vi "DetectElectroMan.vi"(8 "error in (no error)":errorcluster caption="错误输入（无错误）") -> (0 "error out":errorcluster caption="错误输出")   [LabVIEW 2014, in "DetectElectros.lvlib"]
uses:
  DetectElectros.lvlib
  <vilib>/Utility/miscctls.llb/LVRowAndColumnTypeDef.ctl
  DataBase/DataBase.lvlib
panel:
  out "area_name0":string
  out "一行记录":string[](array[string])
  out "结果字符串":string
  in  "OK":bool
  in  "退出":bool
  in  "预览":bool
  in  "清空":bool
  in  "修改":bool
  in  "删除按钮":bool
  in  "添加按钮":bool
  in  "检测电极":i32(listbox)
  in  "填埋区域":i32(listbox)
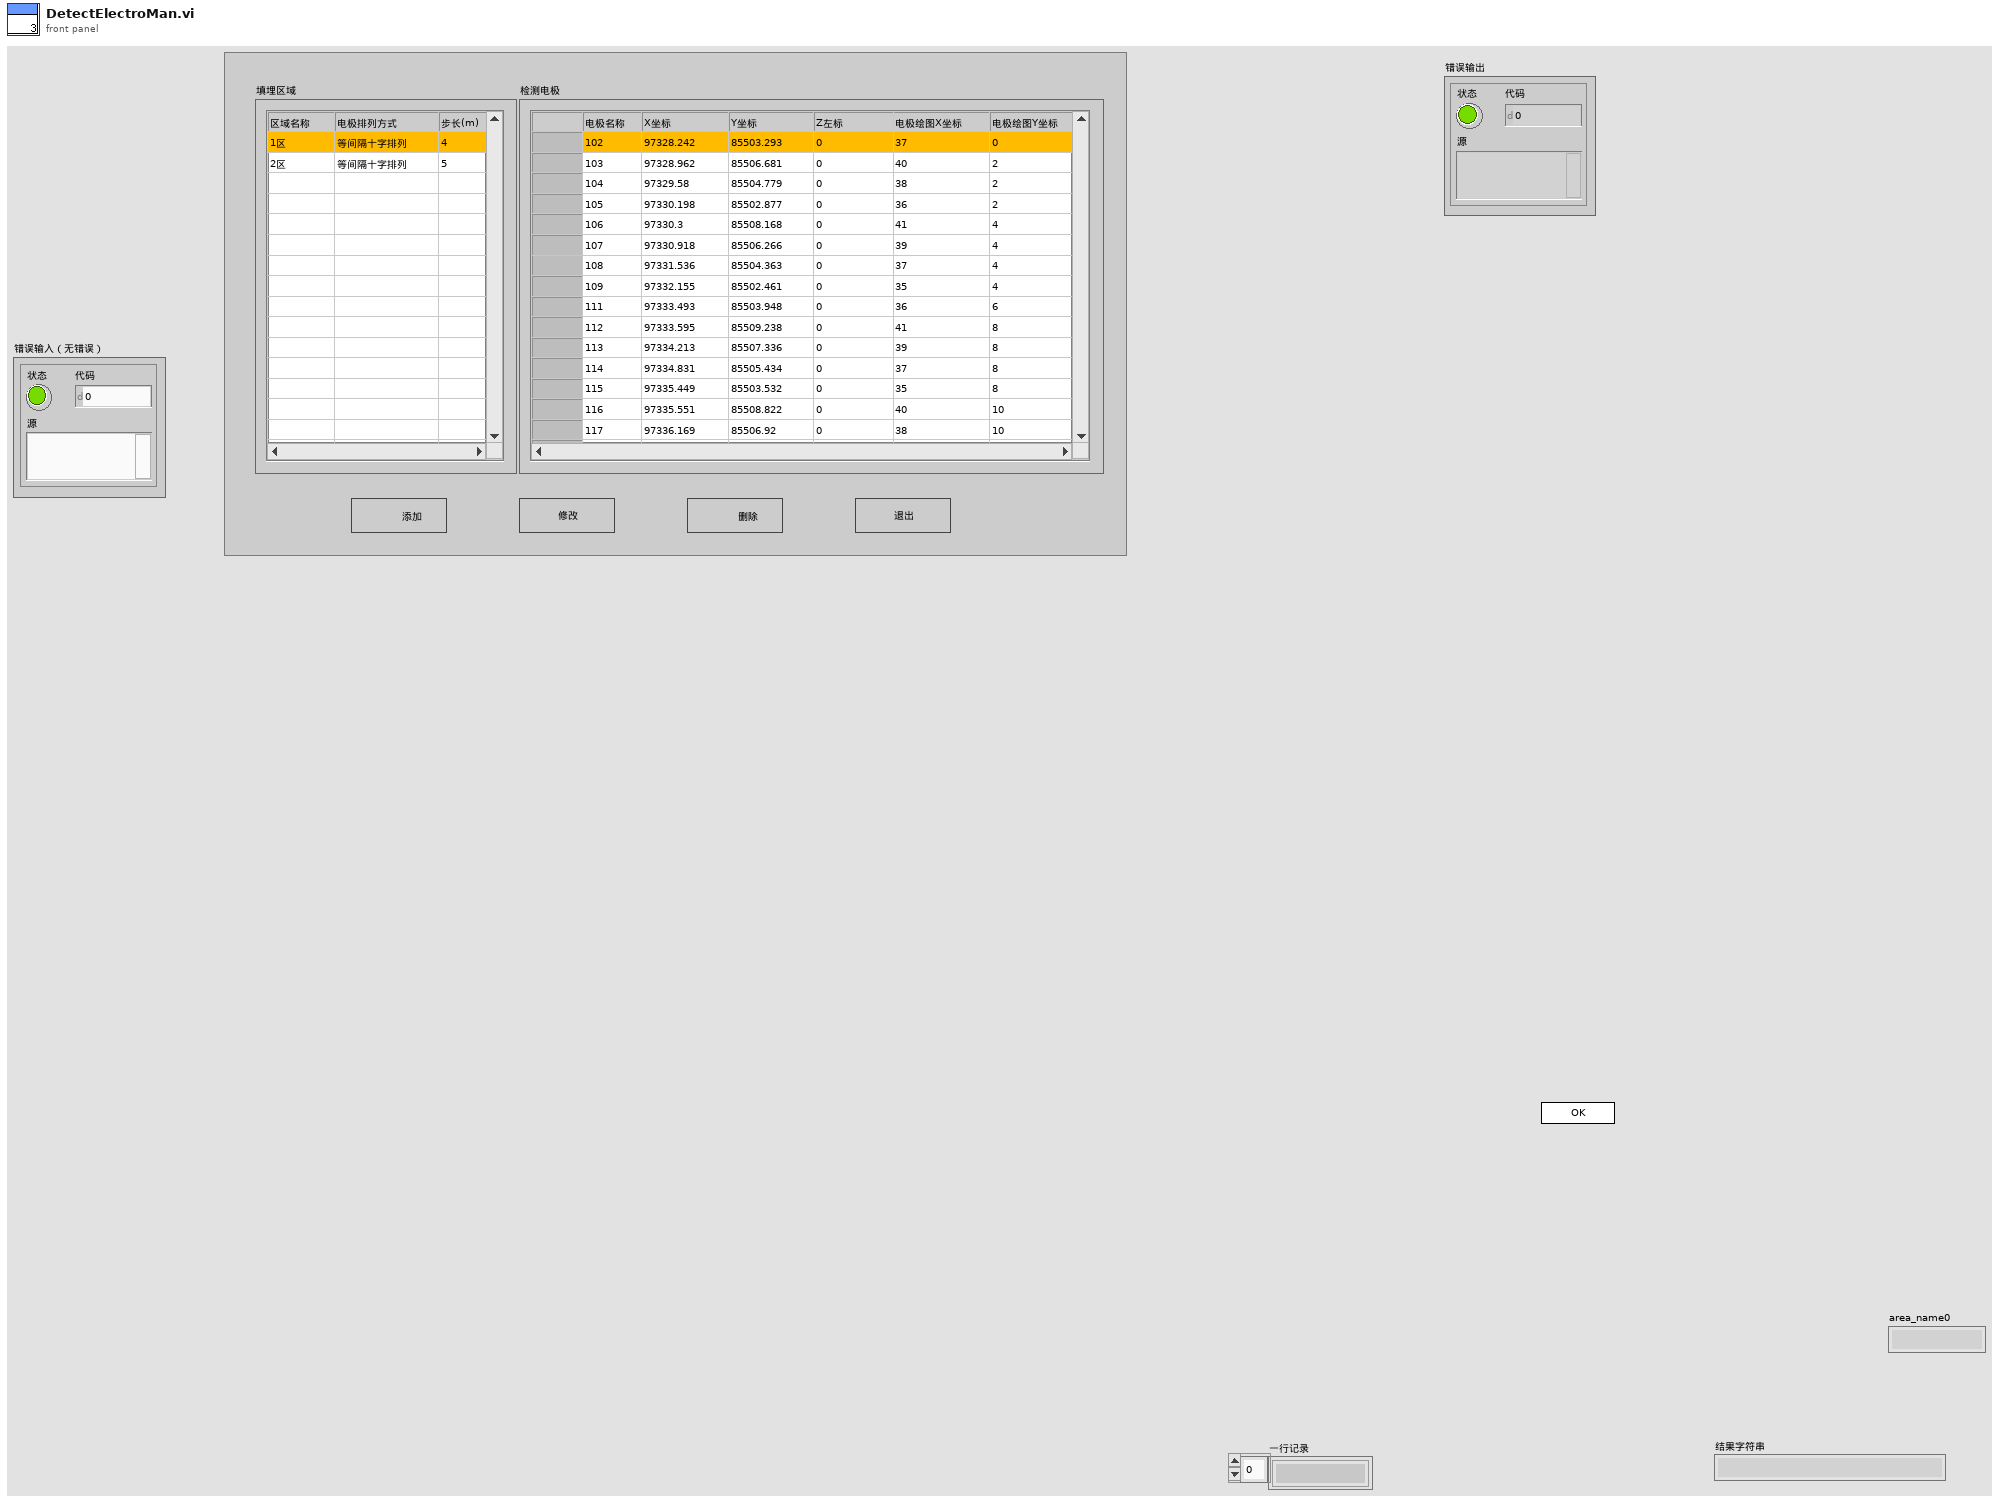
[diagram p1: front panel]
types:
  T1 = enum32{"invalid app kind", "Development System", "Run Time System", "Student Edition", "Embedded LabVIEW", "Evaluation", "Custom"}
  T2 = enum32{"Invalid", "Standard", "Closed", "Hidden", "Minimized", "Maximized"}
  T3 = typedef "LVPoint32TypeDef.ctl" = cluster{"Horizontal":i32, "Vertical":i32}
  T4 = typedef "LVRowAndColumnTypeDef.ctl" = cluster{"Row":i32, "Column":i32}
  T5 = cluster{"Core":cluster{"Current VI Reference":refnum<vi>, "Close Panel on Exit?":bool}, "Your Boolean data":bool, "Your string data":string, "填埋区行列D":T4, "area_name":string, "检测电极行列D":T4}
  T6 = cluster{"Current VI Reference":refnum<vi>, "Close Panel on Exit?":bool}
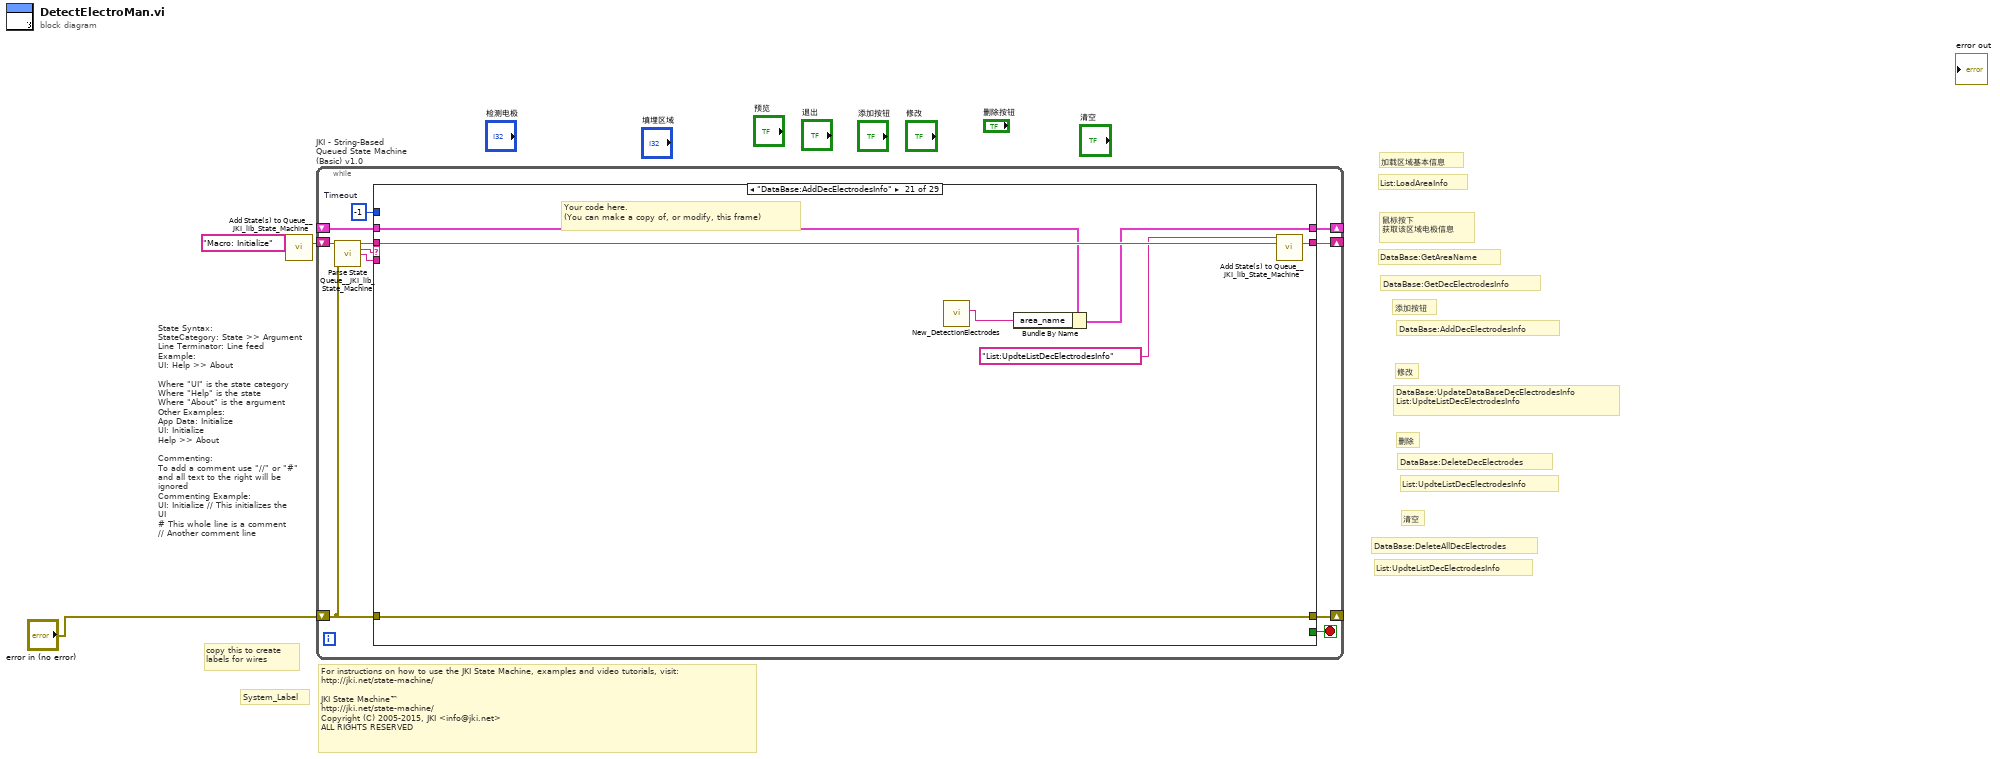
[diagram p0: block diagram]
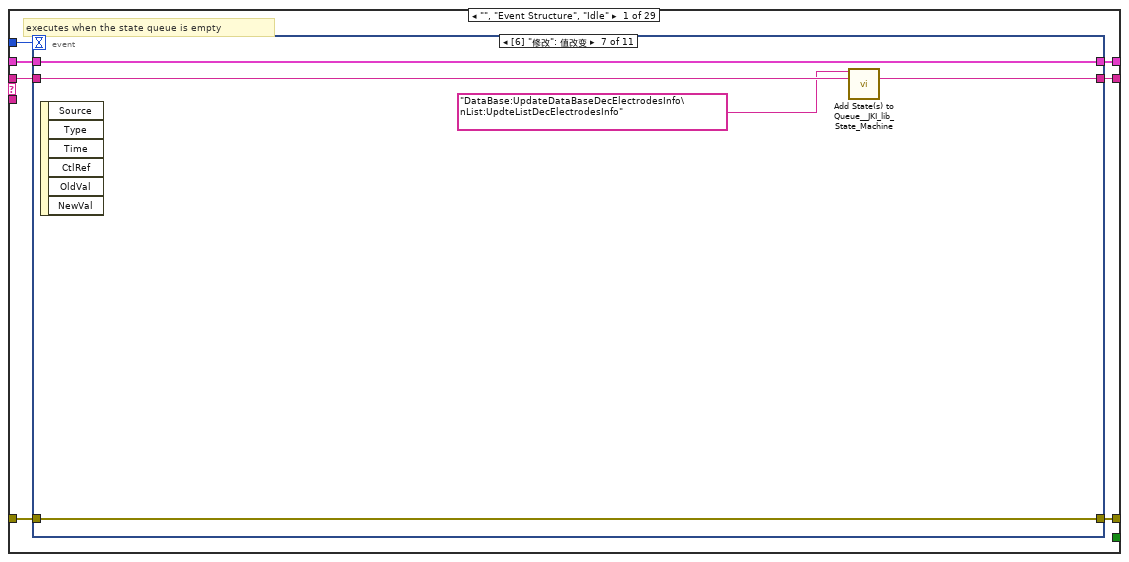
[diagram p2: hidden frame]
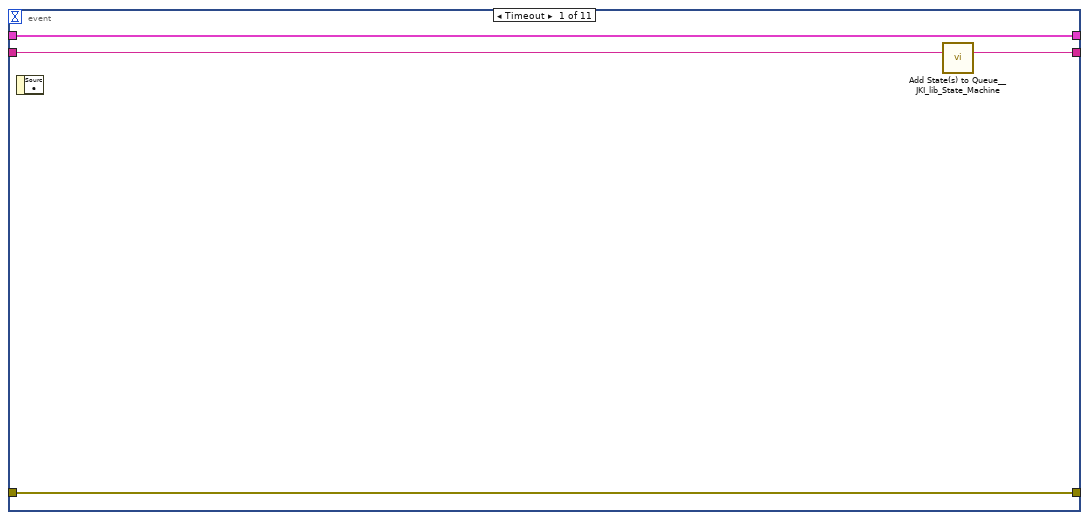
[diagram p3: hidden frame]
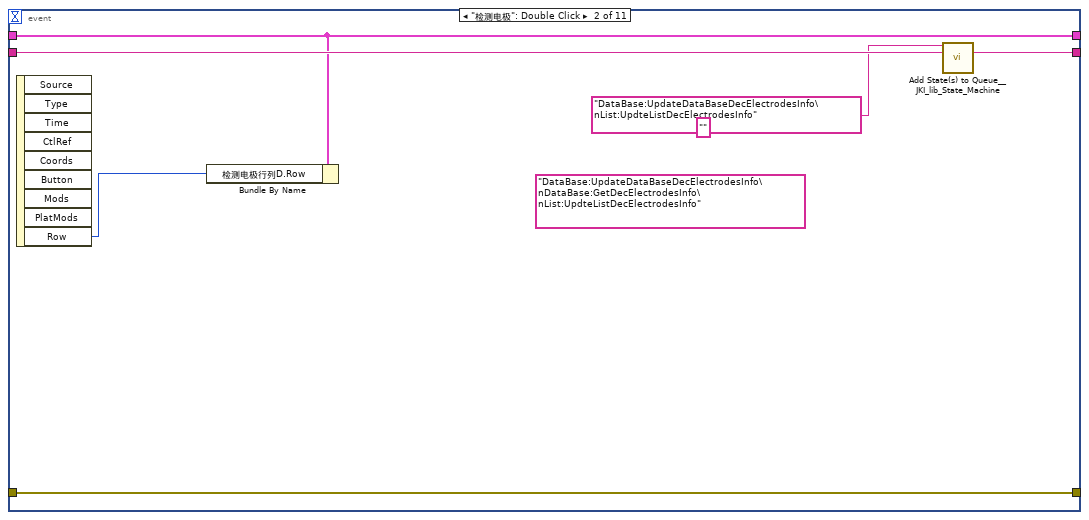
[diagram p4: hidden frame]
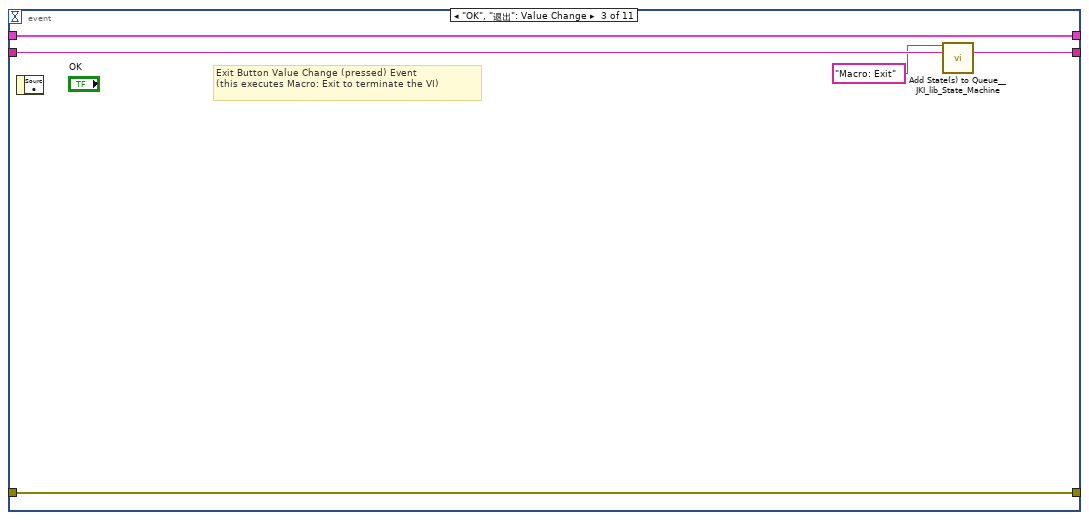
[diagram p5: hidden frame]
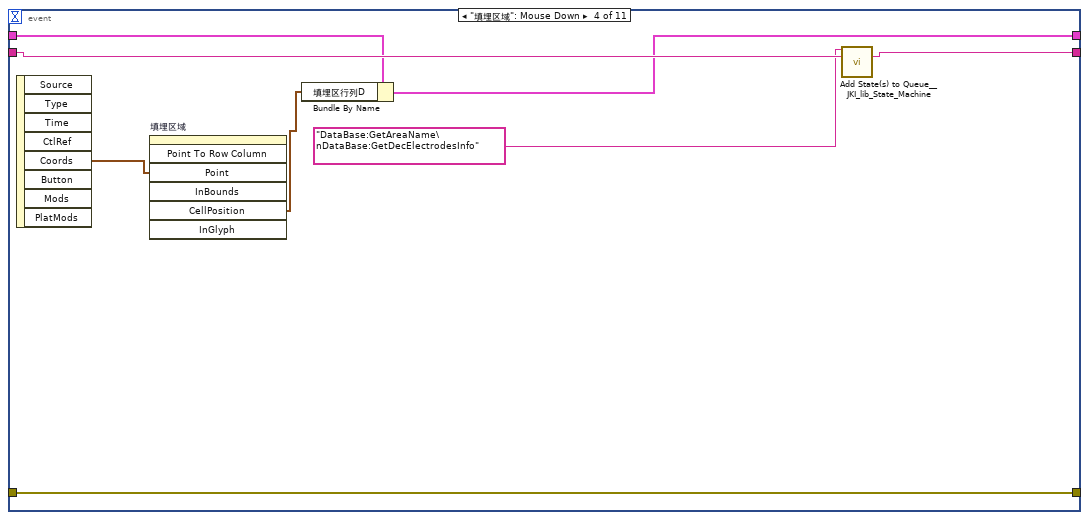
[diagram p6: hidden frame]
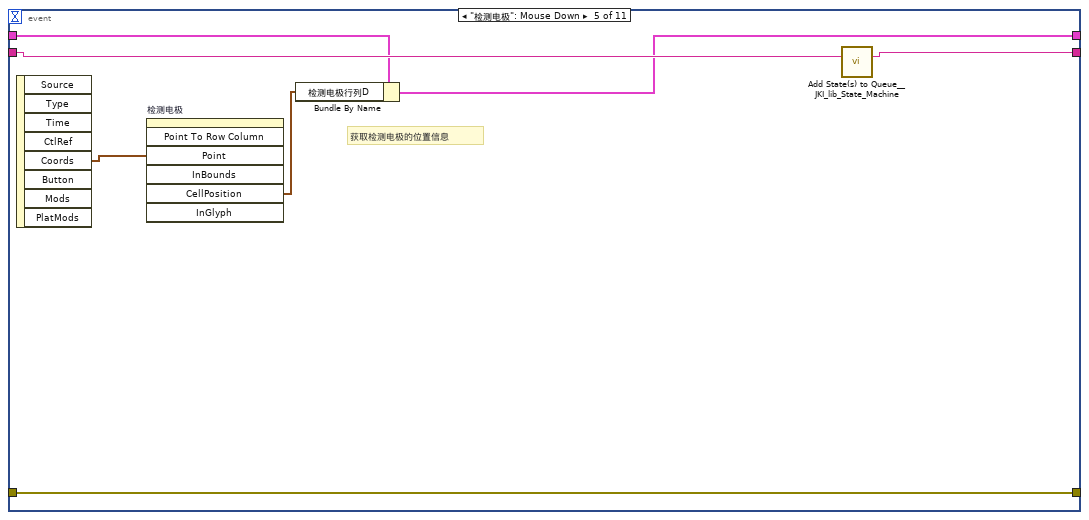
[diagram p7: hidden frame]
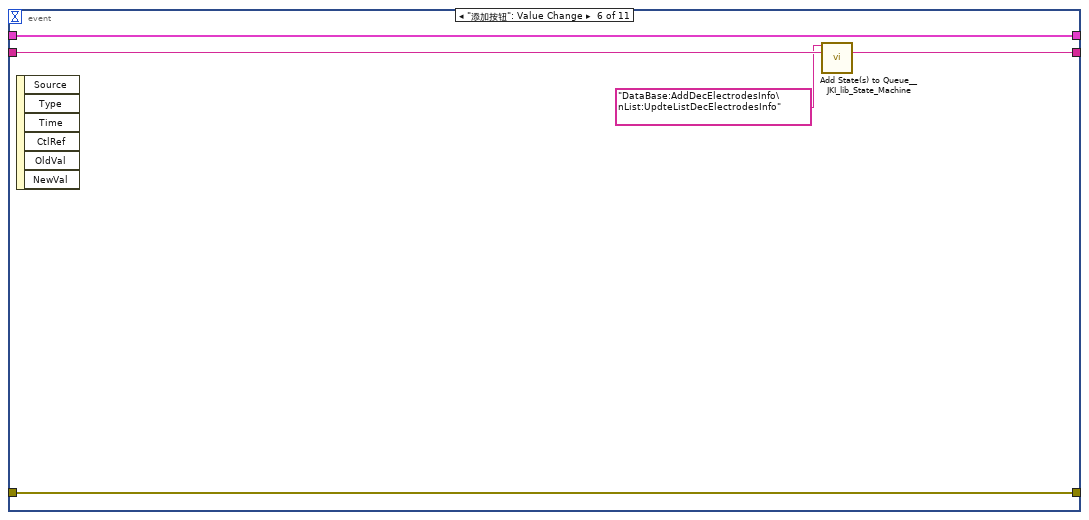
[diagram p8: hidden frame]
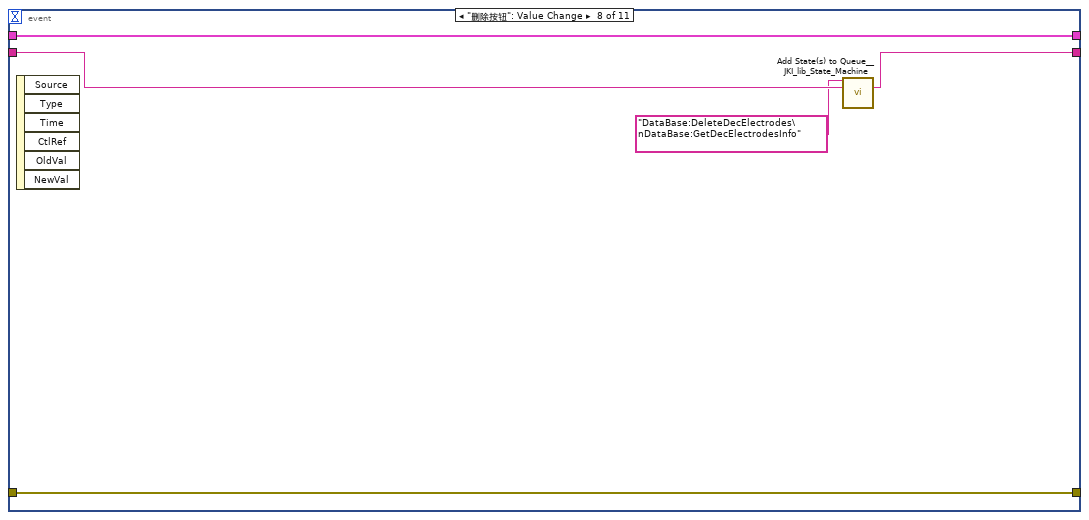
[diagram p9: hidden frame]
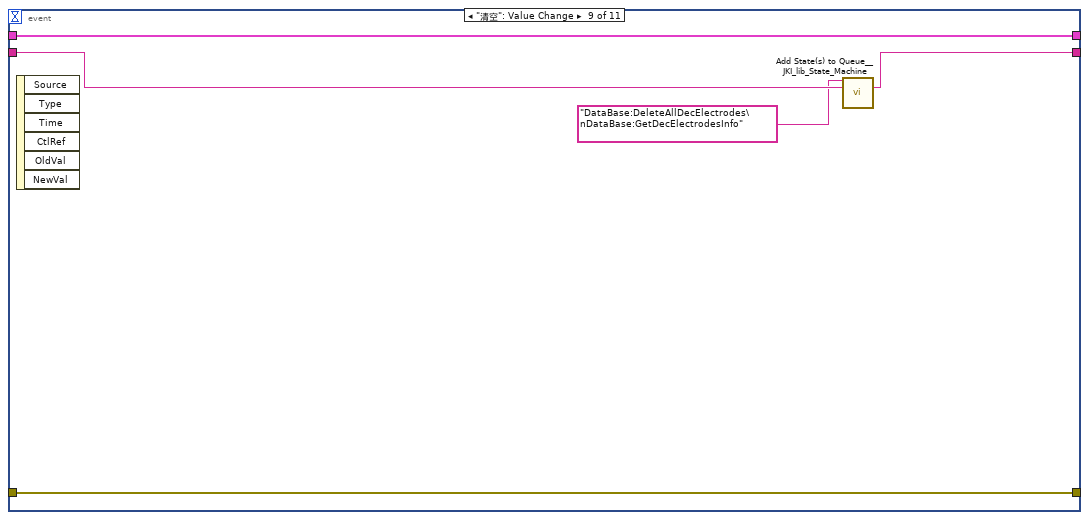
[diagram p10: hidden frame]
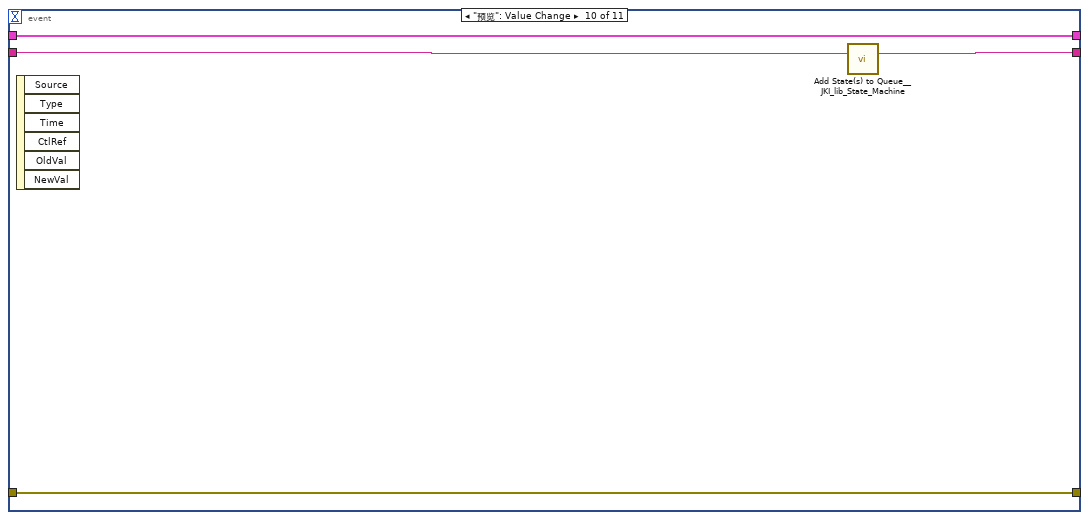
[diagram p11: hidden frame]
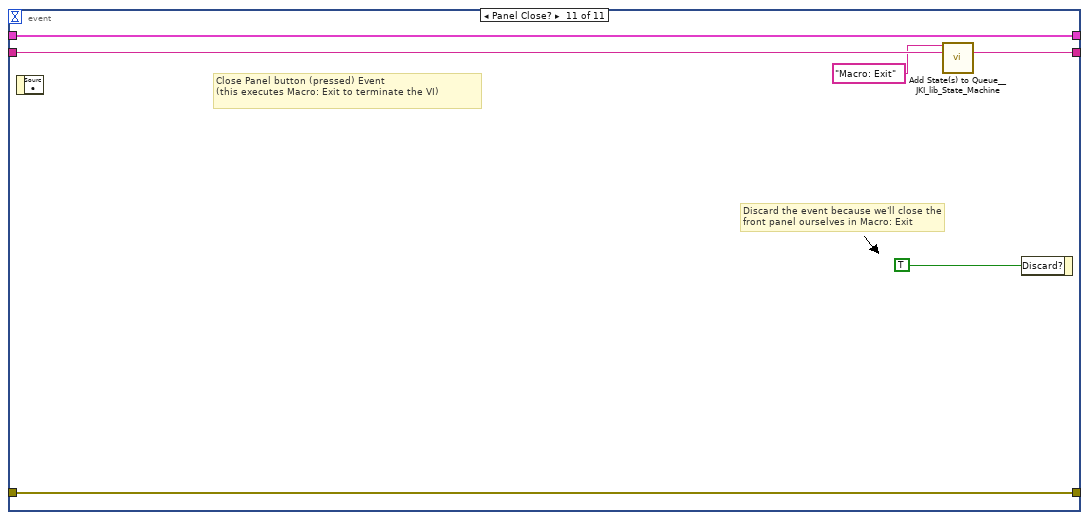
[diagram p12: hidden frame]
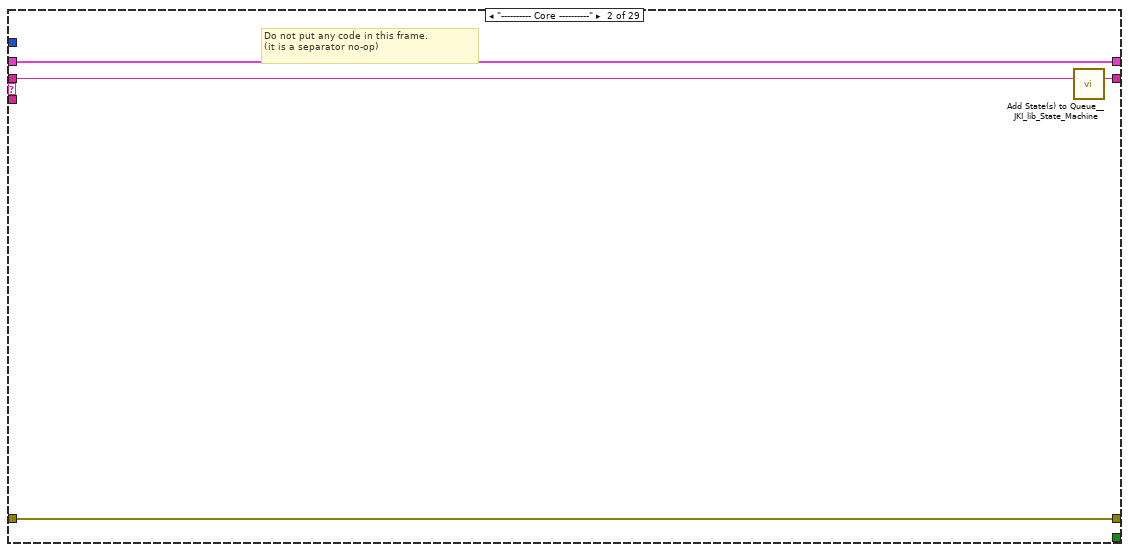
[diagram p13: hidden frame]
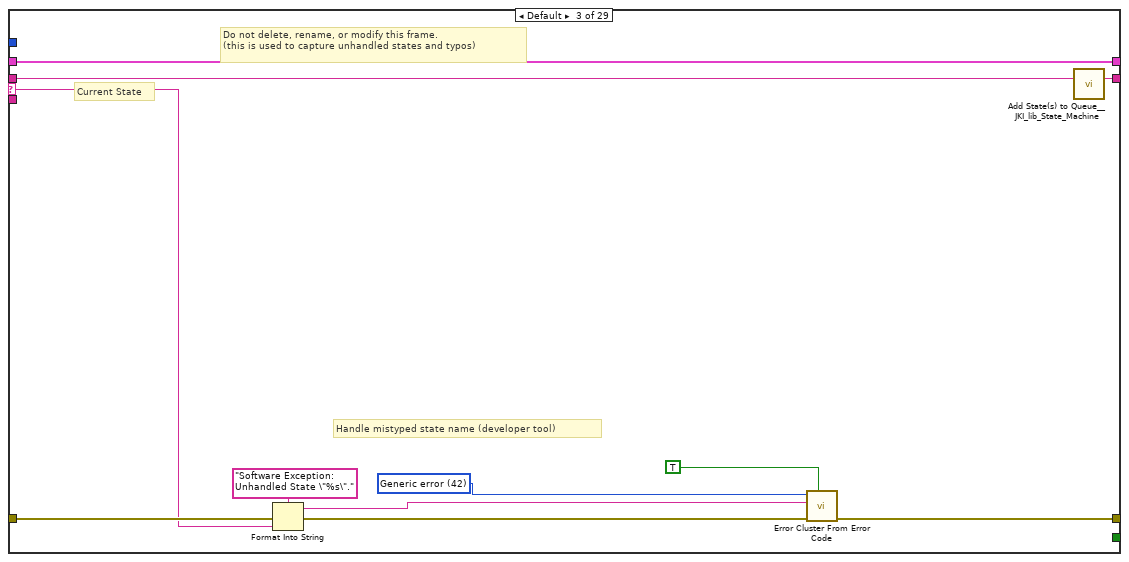
[diagram p14: hidden frame]
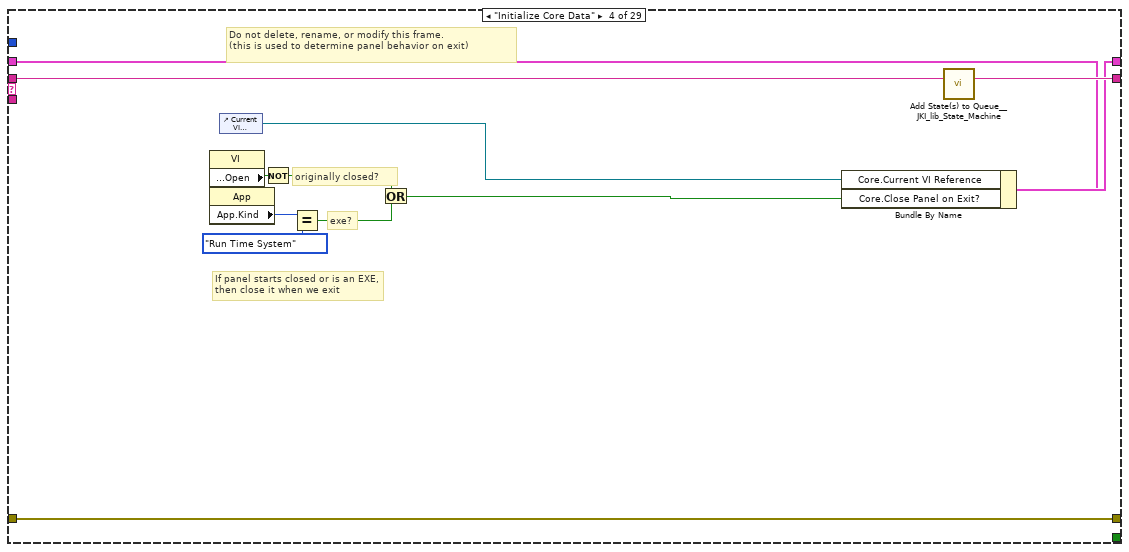
[diagram p15: hidden frame]
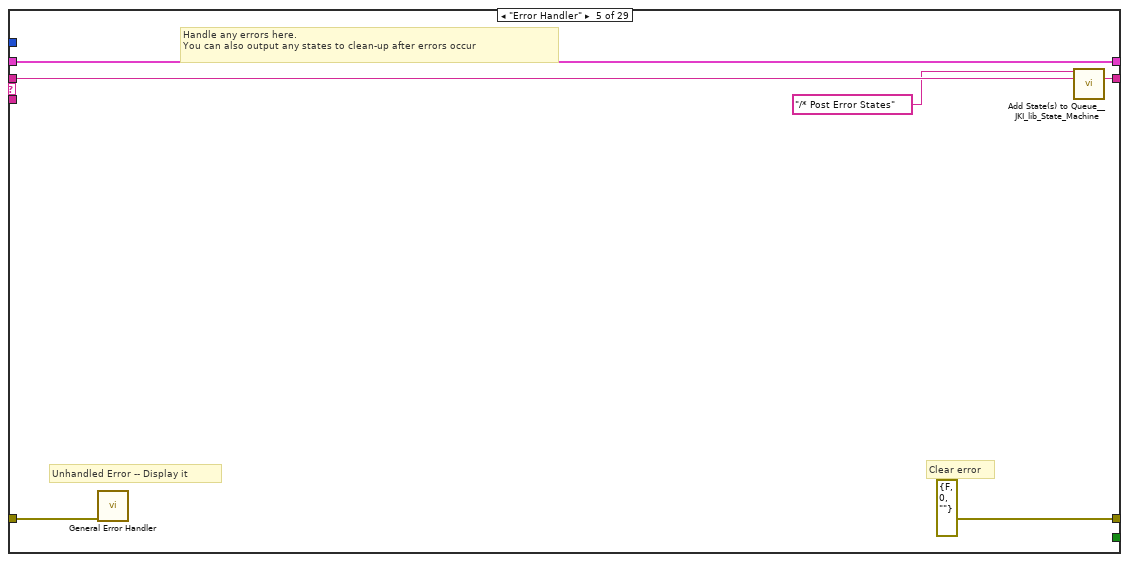
[diagram p16: hidden frame]
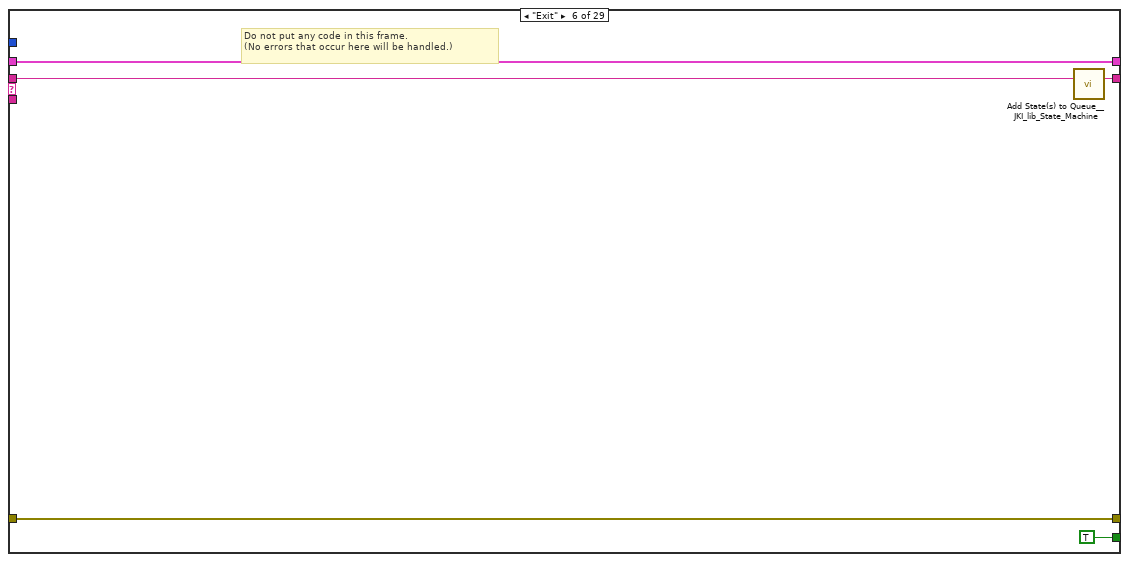
[diagram p17: hidden frame]
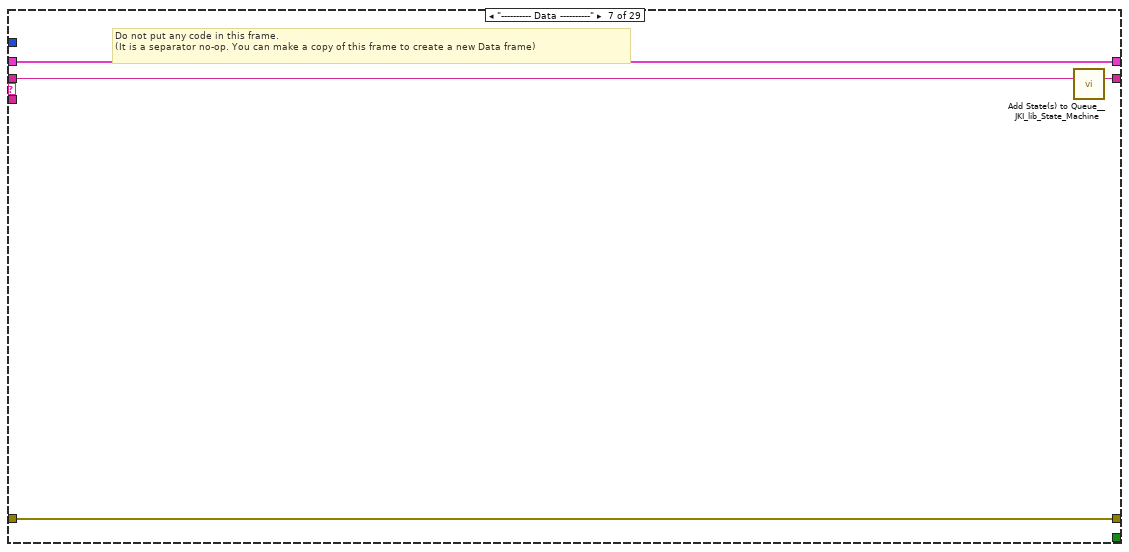
[diagram p18: hidden frame]
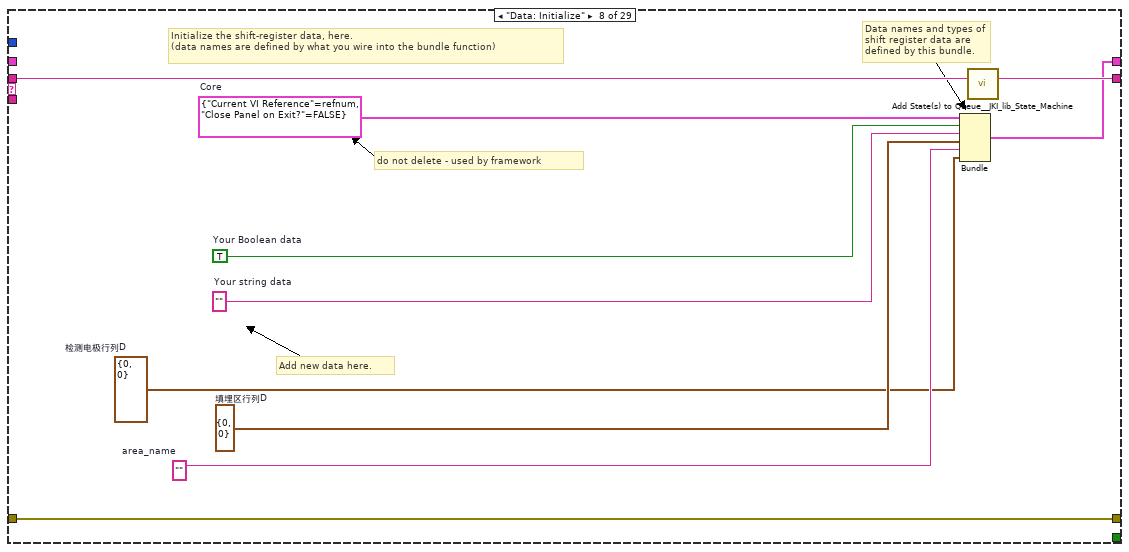
[diagram p19: hidden frame]
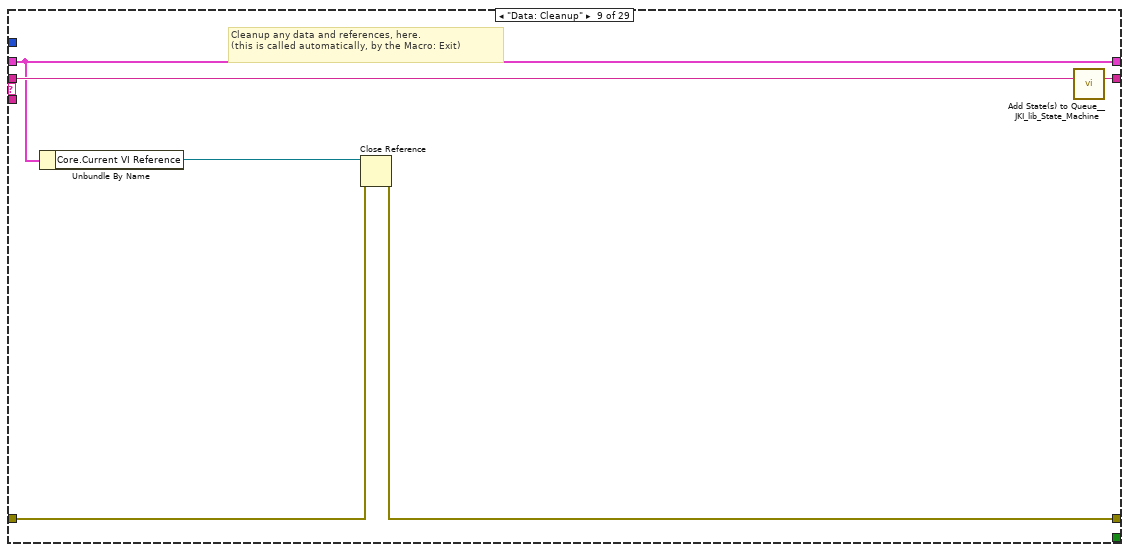
[diagram p20: hidden frame]
diagram:
  # "DataBase:AddDecElectrodesInfo"
  # "添加按钮"
  # "List:UpdteListDecElectrodesInfo"
  # "DataBase:DeleteAllDecElectrodes"
  # "清空"
  # "List:UpdteListDecElectrodesInfo"
  # "DataBase:GetAreaName"
  # "DataBase:DeleteDecElectrodes"
  # "删除"
  # "DataBase:UpdateDataBaseDecElectrodesInfo\nList:UpdteListDecElectrodesInfo"
  # "修改"
  # "DataBase:GetDecElectrodesInfo"
  # "鼠标按下\n获取该区域电极信息"
  # "List:LoadAreaInfo"
  # "加载区域基本信息"
  # "For instructions on how to use the JKI State Machine, examples and video tutorials, visit:\nhttp://jki.net/state-machine/\n\nJKI State Machine™\nhttp://jki.net/state-machine/\nCopyright (C) 2005-2015, JKI <info@jki.net>\nALL RIGHTS RESERVED"
  # "State Syntax:\nStateCategory: State >> Argument\nLine Terminator: Line feed\nExample:\nUI: Help >> About\n\nWhere \"UI\" is the state category\nWhere \"Help\" is the state\nWhere \"About\" is the argument\nOther Examples:\nApp Data: Initialize\nUI: Initialize\nHelp >> About\n\nCommenting:\nTo add a comment use \"//\" or \"#\" and all text to the right will be ignored\nCommenting Example:\nUI: Initialize // This initializes the UI\n# This whole line is a comment\n// Another comment line"
  # "copy this to create labels for wires"
  # "System_Label"
  n1 = call <vilib>:"Add State(s) to Queue__JKI_lib_State_Machine.vi"("State(s) in (\"\")"="Macro: Initialize") -> ("States Out"=w3:string)  [unwired: 14 in]
  n2 = while "JKI - String-Based Queued State Machine (Basic) v1.0" {
    shift-right: [w7] -> _
    shift-left: _ -> [w6]
    shift-right: [w10] -> _
    shift-left: "error in (no error)" -> [w4]
    shift-right: [w9] -> _
    shift-left: w3 -> [w11]
    stop <- w8 stop-if-true
    w5 = -1  # Timeout
    n3 = call <vilib>:"Parse State Queue__JKI_lib_State_Machine.vi"("State Queue"=w11, "Error In (no error)"=w4) -> ("Remaining States"=w13:string, "Current State"=w14:string, "Arguments"=w12:string)  [unwired: 11 in]
    n4 = case shown="\"DataBase:AddDecElectrodesInfo\"" w14 {
      selector: w14 -> [_ _ w86 _ _ _ _ _ _ _ _ _ _ _ _ _ _ _ _ _ _ _ _ _ _ _ _ _ _]
      tunnel: w13 -> [w21 w85 w90 w108 w114 w119 w123 w133 w139 w143 w148 w154 w165 w191 w196 w206 w210 w214 w218 w222 w229 w237 w254 w266 w275 w289 w293 w307 w316]
      tunnel: w12 -> [_ _ _ _ _ _ _ _ _ _ _ w149 w159 _ _ _ _ _ _ _ _ _ _ _ _ _ _ _ _]
      tunnel: w6 -> [w19 w82 w88 w99 w111 w117 w120 _ w134 w140 w146 w152 w161 w188 w193 w203 w207 w211 w215 w219 w225 w232 w239 w259 w268 w277 w290 w295 w313]
      tunnel: [w18 w83 w92 w105 errorcluster {"status"=FALSE, "code"=0, "source"=""} ("error out") w116 w121 w130 w135 w141 w145 w150 w162 w189 w194 w204 w208 w212 w216 w220 w227 w235 w252 w264 w273 w287 w291 w305 w314] -> w10
      tunnel: w4 -> [w17 w83 w91 w105 w110 w116 w121 w130 w136 w141 w145 w151 w163 w189 w194 w204 w208 w212 w216 w220 w227 w235 w252 w264 w273 w287 w291 w305 w314]
      tunnel: [w20 w84 w89 w107 w113 w118 w122 w132 w138 w142 w147 w153 w164 w190 w195 w205 w209 w213 w217 w221 w228 w236 w253 w265 w274 w288 w292 w306 w315] -> w9
      tunnel: [_ _ _ _ _ TRUE _ _ _ _ _ _ _ _ _ _ _ _ _ _ _ _ _ _ _ _ _ _ _] -> w8
      tunnel: [w16 w82 w88 w106 w111 w117 w120 w131 w134 w140 w146 w152 w161 w188 w193 w203 w207 w211 w215 w219 w224 w232 w238 w259 w267 w277 w290 w295 w313] -> w7
      tunnel: w5 -> [w15 _ _ _ _ _ _ _ _ _ _ _ _ _ _ _ _ _ _ _ _ _ _ _ _ _ _ _ _]
      frame "", "Event Structure", "Idle" {
        # "executes when the state queue is empty"
        n5 = event shown="[6] \"修改\": 值改变" {
          selector: _ -> [_ _ _ _ _ _ _ _ _ _ _]
          dyn-events: _ -> [_ _ _ _ _ _ _ _ _ _ _]
          timeout: w15 -> [_ _ _ _ _ _ _ _ _ _ _]
          tunnel: w21 -> [w25 w31 w36 w43 w50 w54 w60 w64 w69 w73 w81]
          tunnel: [w24 w30 w35 w44 w51 w55 w61 w65 w70 w74 w80] -> w20
          tunnel: w19 -> [w22 w28 w33 w39 w48 w56 w58 w66 w71 w75 w78]
          tunnel: [w23 w29 w34 w42 w49 w53 w59 w62 w67 w72 w79] -> w18
          tunnel: w17 -> [w23 w29 w34 w42 w49 w53 w59 w62 w67 w72 w79]
          tunnel: [w22 w28 w33 w38 w47 w56 w58 w66 w71 w75 w78] -> w16
          event Timeout {
            n6 = event-data() -> ()  [unwired: 1 in, 1 out]
            n7 = call <vilib>:"Add State(s) to Queue__JKI_lib_State_Machine.vi"("State(s) in (\"\")"=w25) -> ("States Out"=w24:string)  [unwired: 14 in]
          }
          event "检测电极": Double Click {
            (unwired) "DataBase:UpdateDataBaseDecElectrodesInfo\nDataBase:GetDecElectrodesInfo\nList:UpdteListDecElectrodesInfo"
            (unwired) ""
            n8 = event-data() -> ("Row"=w27:i32)  [unwired: 1 in, 8 out]
            n9 = Bundle By Name(cluster=w28, "检测电极行列D.Row"=w27) -> ()  [unwired: 1 out]
            n10 = call <vilib>:"Add State(s) to Queue__JKI_lib_State_Machine.vi"("State(s) in Front (\"\")"="DataBase:UpdateDataBaseDecElectrodesInfo\nList:UpdteListDecElectrodesInfo", "State(s) in (\"\")"=w31) -> ("States Out"=w30:string)  [unwired: 13 in]
          }
          event "OK", "退出": Value Change {
            # "Exit Button Value Change (pressed) Event\n(this executes Macro: Exit to terminate the VI)"
            n11 = event-data() -> ()  [unwired: 1 in, 1 out]
            n12 = call <vilib>:"Add State(s) to Queue__JKI_lib_State_Machine.vi"("State(s) in Front (\"\")"="Macro: Exit", "State(s) in (\"\")"=w36) -> ("States Out"=w35:string)  [unwired: 13 in]
          }
          event "填埋区域": Mouse Down {
            n13 = event-data() -> ("Coords"=w41:T3)  [unwired: 1 in, 7 out]
            n14 = invoke on="填埋区域" class="MCListbox (严格)" method="Point To Row Column"("Point"=w41) -> ("CellPosition"=w40:T4)  [unwired: 6 in, 6 out]
            n15 = Bundle By Name(cluster=w39, "填埋区行列D"=w40) -> (w38:T5)
            n16 = call <vilib>:"Add State(s) to Queue__JKI_lib_State_Machine.vi"("State(s) in Front (\"\")"="DataBase:GetAreaName\nDataBase:GetDecElectrodesInfo", "State(s) in (\"\")"=w43) -> ("States Out"=w44:string)  [unwired: 13 in]
          }
          event "检测电极": Mouse Down {
            # "获取检测电极的位置信息"
            n17 = event-data() -> ("Coords"=w46:T3)  [unwired: 1 in, 7 out]
            n18 = invoke on="检测电极" class="MCListbox (严格)" method="Point To Row Column"("Point"=w46) -> ("CellPosition"=w45:T4)  [unwired: 6 in, 6 out]
            n19 = Bundle By Name(cluster=w48, "检测电极行列D"=w45) -> (w47:T5)
            n20 = call <vilib>:"Add State(s) to Queue__JKI_lib_State_Machine.vi"("State(s) in (\"\")"=w50) -> ("States Out"=w51:string)  [unwired: 14 in]
          }
          event "添加按钮": Value Change {
            n21 = event-data() -> ()  [unwired: 1 in, 6 out]
            n22 = call <vilib>:"Add State(s) to Queue__JKI_lib_State_Machine.vi"("State(s) in Front (\"\")"="DataBase:AddDecElectrodesInfo\nList:UpdteListDecElectrodesInfo", "State(s) in (\"\")"=w54) -> ("States Out"=w55:string)  [unwired: 13 in]
          }
          event "修改": Value Change {
            n23 = event-data() -> ()  [unwired: 1 in, 6 out]
            n24 = call <vilib>:"Add State(s) to Queue__JKI_lib_State_Machine.vi"("State(s) in Front (\"\")"="DataBase:UpdateDataBaseDecElectrodesInfo\nList:UpdteListDecElectrodesInfo", "State(s) in (\"\")"=w60) -> ("States Out"=w61:string)  [unwired: 13 in]
          }
          event "删除按钮": Value Change {
            n25 = event-data() -> ()  [unwired: 1 in, 6 out]
            n26 = call <vilib>:"Add State(s) to Queue__JKI_lib_State_Machine.vi"("State(s) in Front (\"\")"="DataBase:DeleteDecElectrodes\nDataBase:GetDecElectrodesInfo", "State(s) in (\"\")"=w64) -> ("States Out"=w65:string)  [unwired: 13 in]
          }
          event "清空": Value Change {
            n27 = event-data() -> ()  [unwired: 1 in, 6 out]
            n28 = call <vilib>:"Add State(s) to Queue__JKI_lib_State_Machine.vi"("State(s) in Front (\"\")"="DataBase:DeleteAllDecElectrodes\nDataBase:GetDecElectrodesInfo", "State(s) in (\"\")"=w69) -> ("States Out"=w70:string)  [unwired: 13 in]
          }
          event "预览": Value Change {
            n29 = event-data() -> ()  [unwired: 1 in, 6 out]
            n30 = call <vilib>:"Add State(s) to Queue__JKI_lib_State_Machine.vi"("State(s) in (\"\")"=w73) -> ("States Out"=w74:string)  [unwired: 14 in]
          }
          event Panel Close? {
            # "Discard the event because we'll close the front panel ourselves in Macro: Exit"
            # "Close Panel button (pressed) Event\n(this executes Macro: Exit to terminate the VI)"
            n31 = event-data() -> ()  [unwired: 1 in, 1 out]
            n32 = call <vilib>:"Add State(s) to Queue__JKI_lib_State_Machine.vi"("State(s) in Front (\"\")"="Macro: Exit", "State(s) in (\"\")"=w81) -> ("States Out"=w80:string)  [unwired: 13 in]
            n33 = event-data("Discard?"=TRUE) -> ()  [unwired: 1 in, 1 out]
          }
        }
      }
      frame "---------- Core ----------" {
        # "Do not put any code in this frame.\n(it is a separator no-op)"
        n34 = call <vilib>:"Add State(s) to Queue__JKI_lib_State_Machine.vi"("State(s) in (\"\")"=w85) -> ("States Out"=w84:string)  [unwired: 14 in]
      }
      frame Default {
        w95 = 42 items=["No error", "Argument error", "Memory is full", "Out of zone", "End of file", "File already open", "Generic file I/O error", "File not found", "File permission error", "Disk is full", "Duplicate path", "Too many files open", "System feature not enabled", "Resource file not found", "Cannot add resource", "Resource not found", "Image not found", "Image memory error", "Pen does not exist", "Config type invalid", "Config token not found", "Config parse error", "Config memory error", "Bad external code format", "Bad external code offset", "External code not present", "Null window", "Destroy window error", "Null menu", "Print aborted", "Bad print record", "Print driver error", "Windows error during printing", "Memory error during printing", "Print dialog error", "Generic print error", "Invalid device refnum", "Device not found", "Device parameter error", "Device unit error", "Cannot open device", "Device call aborted", "Generic error", "Cancelled by user", "Object ID too low", "Object ID too high", "Object not in heap", "Unknown heap", "Unknown object (invalid DefProc)", "Unknown object (DefProc not in table)", "Message out of range", "Invalid (null) method", "Unknown message", "Manager call not supported", "Bad address", "Network operation in progress", "Network operation timed out", "Connection is busy", "Network attribute not supported", "Network error", "Address in use", "System out of memory", "Connection aborted", "Connection refused", "Not connected", "Already connected", "Connection closed", "Initialization error (interapplication manager)", "Bad occurrence", "Wait on unbound occurrence handler", "Occurrence queue overflow", "Datalog type conflict", "Unused", "Unrecognized type (interapplication manager)", "Memory corrupt", "Failed to make temporary DLL", "Old CIN version", "Drag socket not found", "Failed to load drop-object", "Failed to register OLE object", "Failed to release OLE object", "Format specifier type mismatch", "Unknown format specifier", "Too few format specifiers", "Too many format specifiers", "Scan failed", "Newer CIN version", "Error converting to variant", "Runtime menu error", "Password tampered", "Variant attribute not found", "Incompatible variant data type", "Event data is not available", "Event Store is not present", "Occurrence is not found", "Event Queue is not created", "Event info is not available", "Refnum passed is NULL", "Error retrieving Class GUID", "Error retrieving CoClass GUID", "Error retrieving TypeLib GUID.", "Bad built application magic bytes.", "Specific driver is different from the specific driver associated with the Logical Name.", "There is no session opened to the class driver.", "Max Error", "MAX - Error with config objects", "MAX - Error loading configuration", "MAX - Group not supported"]
        # "Current State"
        # "Do not delete, rename, or modify this frame.\n(this is used to capture unhandled states and typos)"
        # "Handle mistyped state name (developer tool)"
        n35 = Format Into String(format string="Software Exception: Unhandled State \"%s\"." ("message"), error in=w91, w86) -> (resulting string=w94:string, error out=w93:errorcluster)  [unwired: 1 in]
        n36 = call <vilib>:"Error Cluster From Error Code.vi"("show call chain? (False)"=TRUE, "error in (no error)"=w93, "error message (\"\")"=w94, "error code (0)"=w95) -> ("error out"=w92:errorcluster)  [unwired: 5 in]
        n37 = call <vilib>:"Add State(s) to Queue__JKI_lib_State_Machine.vi"("State(s) in (\"\")"=w90) -> ("States Out"=w89:string)  [unwired: 14 in]
      }
      frame "Initialize Core Data" {
        # "Do not delete, rename, or modify this frame.\n(this is used to determine panel behavior on exit)"
        # "originally closed?"
        # "exe?"
        # "If panel starts closed or is an EXE, then close it when we exit"
        n38 = property class="VI"() -> ("Front Panel.Open"=w104:bool)  [unwired: 2 in, 2 out]
        n39 = property class="App"() -> ("App.Kind"=w103:T1)  [unwired: 2 in, 2 out]
        n40 = control-ref of="Current VI Reference"() -> (w97:refnum<vi>)
        n41 = Not(x=w104) -> (.not. x?=w101:bool)
        n42 = Equal?(x=w103, y=T1."Run Time System" ("Application:Kind")) -> (x = y?=w100:bool)
        n43 = Or(x=w101, y=w100) -> (x .or. y?=w98:bool)
        n44 = Bundle By Name(cluster=w99, "Core.Current VI Reference"=w97, "Core.Close Panel on Exit?"=w98) -> (w106:T5)
        n45 = call <vilib>:"Add State(s) to Queue__JKI_lib_State_Machine.vi"("State(s) in (\"\")"=w108) -> ("States Out"=w107:string)  [unwired: 14 in]
      }
      frame "Error Handler" {
        # "Unhandled Error -- Display it"
        # "Handle any errors here.\nYou can also output any states to clean-up after errors occur"
        # "Clear error"
        n46 = call <vilib>:"General Error Handler.vi"("error in (no error)"=w110) -> ()  [unwired: 10 in, 5 out]
        n47 = call <vilib>:"Add State(s) to Queue__JKI_lib_State_Machine.vi"("State(s) in Front (\"\")"="/* Post Error States", "State(s) in (\"\")"=w114) -> ("States Out"=w113:string)  [unwired: 13 in]
      }
      frame "Exit" {
        # "Do not put any code in this frame.\n(No errors that occur here will be handled.)"
        n48 = call <vilib>:"Add State(s) to Queue__JKI_lib_State_Machine.vi"("State(s) in (\"\")"=w119) -> ("States Out"=w118:string)  [unwired: 14 in]
      }
      frame "---------- Data ----------" {
        # "Do not put any code in this frame.\n(It is a separator no-op. You can make a copy of this frame to create a new Data frame)"
        n49 = call <vilib>:"Add State(s) to Queue__JKI_lib_State_Machine.vi"("State(s) in (\"\")"=w123) -> ("States Out"=w122:string)  [unwired: 14 in]
      }
      frame "Data: Initialize" {
        w124 = T4 {"Row"=0, "Column"=0}  # 检测电极行列D
        w125 = ""  # area_name
        w126 = T4 {"Row"=0, "Column"=0}  # 填埋区行列D
        w127 = T6 {"Current VI Reference"=refnum, "Close Panel on Exit?"=FALSE}  # Core
        w129 = TRUE  # Your Boolean data
        w128 = ""  # Your string data
        # "do not delete - used by framework"
        # "Add new data here."
        # "Data names and types of shift register data are defined by this bundle."
        # "Initialize the shift-register data, here.\n(data names are defined by what you wire into the bundle function)"
        n50 = Bundle("Core"=w127, "Your Boolean data"=w129, "Your string data"=w128, "填埋区行列D"=w126, "area_name"=w125, "检测电极行列D"=w124) -> (w131:T5)  [unwired: 1 in]
        n51 = call <vilib>:"Add State(s) to Queue__JKI_lib_State_Machine.vi"("State(s) in (\"\")"=w133) -> ("States Out"=w132:string)  [unwired: 14 in]
      }
      frame "Data: Cleanup" {
        # "Cleanup any data and references, here.\n(this is called automatically, by the Macro: Exit)"
        n52 = Unbundle By Name(w134) -> ("Core.Current VI Reference"=w137:refnum<vi>)
        n53 = Close Reference(reference=w137, error in (no error)=w136) -> (error out=w135:errorcluster)
        n54 = call <vilib>:"Add State(s) to Queue__JKI_lib_State_Machine.vi"("State(s) in (\"\")"=w139) -> ("States Out"=w138:string)  [unwired: 14 in]
      }
      frame "---------- UI ----------" {
        # "Do not put any code in this frame.\n(It is a separator no-op. You can make a copy of this frame to create a new UI frame)"
        n55 = call <vilib>:"Add State(s) to Queue__JKI_lib_State_Machine.vi"("State(s) in (\"\")"=w143) -> ("States Out"=w142:string)  [unwired: 14 in]
      }
      frame "UI: Initialize" {
        # "Initialize the User Interface, here.\n(this is called automatically, by the Macro: Init)"
        n56 = call <vilib>:"Add State(s) to Queue__JKI_lib_State_Machine.vi"("State(s) in Front (\"\")"="List:LoadAreaInfo", "State(s) in (\"\")"=w148) -> ("States Out"=w147:string)  [unwired: 13 in]
      }
      frame "UI: Cursor Set" {
        # "Argument"
        # "Set and Unset Cursor Busy.\n(Usage: \"UI: Cursor Set >> Busy|Idle\")"
        n57 = case shown="\"Idle\", 默认" w149 {
          tunnel: w151 -> [w156 w158]
          tunnel: [w155 w157] -> w150
          frame "Idle", Default {
            n58 = call <vilib>:"Unset Busy.vi"("error in (no error)"=w156) -> ("error out"=w155:errorcluster)  [unwired: 10 in]
          }
          frame "Busy" {
            n59 = call <vilib>:"Set Busy.vi"("error in (no error)"=w158) -> ("error out"=w157:errorcluster)  [unwired: 9 in, 1 out]
          }
        }
        n60 = call <vilib>:"Add State(s) to Queue__JKI_lib_State_Machine.vi"("State(s) in (\"\")"=w154) -> ("States Out"=w153:string)  [unwired: 14 in]
      }
      frame "UI: Front Panel State" {
        # "Argument"
        # "Set Front Panel Open or Closed\n(Usage: \"UI: Front Panel State >> Open|Close\")"
        n61 = Unbundle By Name(w161) -> ("Core.Current VI Reference"=w160:refnum<vi>)
        n62 = case shown="\"Open\", 默认" w159 {
          tunnel: w163 -> [w169 w182]
          tunnel: [w171 w183] -> w162
          tunnel: w160 -> [w170 w180]
          frame "Open", Default {
            n63 = property class="VI"(reference=w170, error in=w169) -> (reference out=w167:refnum<vi>, error out=w168:errorcluster, "Front Panel.Open"=w166:bool)
            n64 = case shown="假" w166 {
              tunnel: [w174 w177] -> w171
              tunnel: w168 -> [w173 w177]
              tunnel: w167 -> [w172 _]
              frame False {
                n65 = invoke class="VI" method="FP.Open"(reference=w172, error in=w173, "Activate"=TRUE, "State"=T2."Standard") -> (error out=w174:errorcluster)  [unwired: 1 in, 4 out]
              }
              frame True {
              }
            }
          }
          frame "Close" {
            n66 = property class="VI"(reference=w180, error in=w182) -> (reference out=w179:refnum<vi>, error out=w181:errorcluster, "Front Panel.Open"=w178:bool)
            n67 = case shown="真" w178 {
              tunnel: [w184 w187] -> w183
              tunnel: w181 -> [w184 w186]
              tunnel: w179 -> [_ w185]
              frame False {
              }
              frame True {
                n68 = invoke class="VI" method="FP.Close"(reference=w185, error in=w186) -> (error out=w187:errorcluster)  [unwired: 1 in, 2 out]
              }
            }
          }
        }
        n69 = call <vilib>:"Add State(s) to Queue__JKI_lib_State_Machine.vi"("State(s) in (\"\")"=w165) -> ("States Out"=w164:string)  [unwired: 14 in]
      }
      frame "---------- Macro ----------" {
        # "Do not put any code in this frame.\n(It is a separator no-op. You can make a copy of this frame to create a new Macro frame)"
        n70 = call <vilib>:"Add State(s) to Queue__JKI_lib_State_Machine.vi"("State(s) in (\"\")"=w191) -> ("States Out"=w190:string)  [unwired: 14 in]
      }
      frame "Macro: Initialize" {
        w192 = "Data: Initialize\nInitialize Core Data\nUI: Initialize\nUI: Front Panel State >> Open"  # Data: Initialize Initialize Core Data UI: Initialize UI: Front Panel State >> Open
        # "Initialization Macro\n(This is called once, when the VI starts)"
        n71 = call <vilib>:"Add State(s) to Queue__JKI_lib_State_Machine.vi"("State(s) in Front (\"\")"=w192, "State(s) in (\"\")"=w196) -> ("States Out"=w195:string)  [unwired: 13 in]
      }
      frame "Macro: Exit" {
        # "Exit Macro\n(This is called once, when the VI exits)"
        n72 = Unbundle By Name(w203) -> ("Core.Close Panel on Exit?"=w202:bool)
        n73 = Select(t="UI: Front Panel State >> Close", s=w202, f="") -> (s? t:f=w199:string)
        n74 = call <vilib>:"Add State(s) to Queue__JKI_lib_State_Machine.vi"("State(s) in (\"\")"=w199, "State(s) at Back (\"\")"="Data: Cleanup\nExit") -> ("States Out"=w197:string)  [unwired: 13 in]
        n75 = call <vilib>:"Add State(s) to Queue__JKI_lib_State_Machine.vi"("State(s) in Front (\"\")"=w197, "State(s) in (\"\")"=w206) -> ("States Out"=w205:string)  [unwired: 13 in]
      }
      frame "---------- New Category ----------" {
        # "Template Separator\n(You can make a copy of, or modify, this frame)"
        n76 = call <vilib>:"Add State(s) to Queue__JKI_lib_State_Machine.vi"("State(s) in (\"\")"=w210) -> ("States Out"=w209:string)  [unwired: 14 in]
      }
      frame "New Category: 1" {
        # "Your code here.\n(You can make a copy of, or modify, this frame)"
        n77 = call <vilib>:"Add State(s) to Queue__JKI_lib_State_Machine.vi"("State(s) in (\"\")"=w214) -> ("States Out"=w213:string)  [unwired: 14 in]
      }
      frame "New Category: 2" {
        # "Your code here.\n(You can make a copy of, or modify, this frame)"
        n78 = call <vilib>:"Add State(s) to Queue__JKI_lib_State_Machine.vi"("State(s) in (\"\")"=w218) -> ("States Out"=w217:string)  [unwired: 14 in]
      }
      frame "----------DataBase----------" {
        # "Your code here.\n(You can make a copy of, or modify, this frame)"
        n79 = call <vilib>:"Add State(s) to Queue__JKI_lib_State_Machine.vi"("State(s) in (\"\")"=w222) -> ("States Out"=w221:string)  [unwired: 14 in]
      }
      frame "DataBase:AddDecElectrodesInfo" {
        # "Your code here.\n(You can make a copy of, or modify, this frame)"
        n80 = call "New_DetectionElectrodes.vi"() -> ("AreaName"=w226:string)  [unwired: 11 in]
        n81 = Bundle By Name(cluster=w225, "area_name"=w226) -> (w224:T5)
        n82 = call <vilib>:"Add State(s) to Queue__JKI_lib_State_Machine.vi"("State(s) in Front (\"\")"="List:UpdteListDecElectrodesInfo", "State(s) in (\"\")"=w229) -> ("States Out"=w228:string)  [unwired: 13 in]
      }
      frame "DataBase:DeleteAllDecElectrodes" {
        # "Your code here.\n(You can make a copy of, or modify, this frame)"
        n83 = Unbundle By Name(w232) -> ("area_name"=w231:string)
        n84 = Format Into String(format string="delete from t_detection_electrodes where  area_name='%s';", w231) -> (resulting string=w234:string)  [unwired: 2 in, 1 out]
        n85 = call "deleteData.vi"("SQL query"=w234) -> ()  [unwired: 10 in, 1 out]
        n86 = call <vilib>:"Add State(s) to Queue__JKI_lib_State_Machine.vi"("State(s) in Front (\"\")"="List:UpdteListDecElectrodesInfo", "State(s) in (\"\")"=w237) -> ("States Out"=w236:string)  [unwired: 13 in]
      }
      frame "DataBase:GetAreaName" {
        # "Your code here.\n(You can make a copy of, or modify, this frame)"
        n87 = Unbundle By Name(w239) -> ("填埋区行列D.Row"=w251:i32)
        n88 = Absolute Value(x=w251) -> (abs(x)=w242:i32)
        n89 = Number To Decimal String(number=w242) -> (decimal integer string=w248:string)  [unwired: 1 in]
        n90 = Format Into String(format string="select area_name from t_area limit %s,1;", w248) -> (resulting string=w249:string, error out=w247:errorcluster)  [unwired: 2 in]
        "结果字符串" <- w249
        n91 = call "SelectData.vi"("SQL query"=w249, "error in"=w247) -> ("recordset data"=w246:variant[][])  [unwired: 6 in, 1 out]
        n92 = call "ReadDataFromDatabase.vi"("长度"=1, "index"=0, "recordset data"=w246) -> ("一行记录"=w243:string[])  [unwired: 7 in, 1 out]
        "一行记录" <- w243
        n93 = Index Array(array=w243, index=0 ("索引")) -> (element=w240:string)
        "area_name0" <- w240
        n94 = Bundle By Name(cluster=w239, "area_name"=w240) -> (w238:T5)
        n95 = call <vilib>:"Add State(s) to Queue__JKI_lib_State_Machine.vi"("State(s) in (\"\")"=w254) -> ("States Out"=w253:string)  [unwired: 14 in]
      }
      frame "DataBase:DeleteDecElectrodes" {
        # "Your code here.\n(You can make a copy of, or modify, this frame)"
        n96 = Unbundle By Name(w259) -> ("检测电极行列D.Row"=w263:i32)
        n97 = Unbundle By Name(w259) -> ("area_name"=w258:string)
        n98 = Absolute Value(x=w263) -> (abs(x)=w261:i32)
        n99 = Number To Decimal String(number=w261) -> (decimal integer string=w260:string)  [unwired: 1 in]
        n100 = Format Into String(format string="delete from t_detection_electrodes where  detection_electrodes_id=(select td.detection_electrodes_id from (select detection_electrodes_id from t_detection_electrodes where  area_name='%s' limit %s,1) td);", w258, w260) -> (resulting string=w257:string, error out=w256:errorcluster)  [unwired: 2 in]
        n101 = call "deleteData.vi"("error in"=w256, "SQL query"=w257) -> ()  [unwired: 9 in, 1 out]
        n102 = call <vilib>:"Add State(s) to Queue__JKI_lib_State_Machine.vi"("State(s) in Front (\"\")"="List:UpdteListDecElectrodesInfo", "State(s) in (\"\")"=w266) -> ("States Out"=w265:string)  [unwired: 13 in]
      }
      frame "DataBase:UpdateDataBaseDecElectrodesInfo" {
        (unwired) "List:UpdteListDecElectrodesInfo"
        # "Your code here.\n(You can make a copy of, or modify, this frame)"
        n103 = Unbundle By Name(w268) -> ("area_name"=w270:string)
        n104 = Unbundle By Name(w268) -> ("检测电极行列D.Row"=w272:i32)
        n105 = Absolute Value(x=w272) -> (abs(x)=w271:i32)
        n106 = call "Modify_DetectionElectrodes.vi"("序号"=w271, "区域名称"=w270) -> ("out区域名称"=w269:string)  [unwired: 7 in, 2 out]
        n107 = Bundle By Name(cluster=w268, "area_name"=w269) -> (w267:T5)
        n108 = call <vilib>:"Add State(s) to Queue__JKI_lib_State_Machine.vi"("State(s) in (\"\")"=w275) -> ("States Out"=w274:string)  [unwired: 14 in]
      }
      frame "DataBase:GetDecElectrodesInfo" {
        # "Your code here.\n(You can make a copy of, or modify, this frame)"
        n109 = Unbundle By Name(w277) -> ("area_name"=w276:string)
        n110 = Format Into String(format string="select * from t_detection_electrodes where area_name='%s';", w276) -> (resulting string=w285:string)  [unwired: 2 in, 1 out]
        n111 = call "SelectData.vi"("SQL query"=w285) -> ("recordset data"=w284:variant[][])  [unwired: 7 in, 1 out]
        n112 = call "ReadDataFromDatabase.vi"("长度"=8, "index"=1, "recordset data"=w284) -> ("所有记录"=w281:string[][])  [unwired: 7 in, 1 out]
        n113 = Delete From Array(array=w281, length=1 ("长度"), index (col)=1 ("禁用的索引 (列)")) -> (array with subset deleted=w278:string[][])  [unwired: 1 in, 1 out]
        n114 = property on="检测电极" class="MCListbox (严格)"("ItemNames"=w278) -> ()  [unwired: 2 in, 2 out]
        n115 = call <vilib>:"Add State(s) to Queue__JKI_lib_State_Machine.vi"("State(s) in (\"\")"=w289) -> ("States Out"=w288:string)  [unwired: 14 in]
      }
      frame "------List-----" {
        # "Your code here.\n(You can make a copy of, or modify, this frame)"
        n116 = call <vilib>:"Add State(s) to Queue__JKI_lib_State_Machine.vi"("State(s) in (\"\")"=w293) -> ("States Out"=w292:string)  [unwired: 14 in]
      }
      frame "List:UpdteListDecElectrodesInfo" {
        # "Your code here.\n(You can make a copy of, or modify, this frame)"
        n117 = Unbundle By Name(w295) -> ("area_name"=w294:string)
        n118 = Format Into String(format string="select * from t_detection_electrodes where area_name='%s';", w294) -> (resulting string=w303:string)  [unwired: 2 in, 1 out]
        n119 = call "SelectData.vi"("SQL query"=w303) -> ("recordset data"=w296:variant[][])  [unwired: 7 in, 1 out]
        n120 = call "ReadDataFromDatabase.vi"("长度"=8, "index"=1, "recordset data"=w296) -> ("所有记录"=w299:string[][])  [unwired: 7 in, 1 out]
        n121 = Delete From Array(array=w299, length=1 ("长度"), index (col)=1 ("禁用的索引 (列)")) -> (array with subset deleted=w304:string[][])  [unwired: 1 in, 1 out]
        n122 = property on="检测电极" class="MCListbox (严格)"("ItemNames"=w304) -> ()  [unwired: 2 in, 2 out]
        n123 = call <vilib>:"Add State(s) to Queue__JKI_lib_State_Machine.vi"("State(s) in (\"\")"=w307) -> ("States Out"=w306:string)  [unwired: 14 in]
      }
      frame "List:LoadAreaInfo" {
        # "Your code here.\n(You can make a copy of, or modify, this frame)"
        n124 = call "SelectData.vi"("SQL query"="select *from t_area;") -> ("recordset data"=w311:variant[][])  [unwired: 7 in, 1 out]
        n125 = call "ReadDataFromDatabase.vi"("长度"=3, "index"=1, "recordset data"=w311) -> ("所有记录"=w309:string[][])  [unwired: 7 in, 1 out]
        n126 = property on="填埋区域" class="MCListbox (严格)"("ItemNames"=w309) -> ()  [unwired: 2 in, 2 out]
        n127 = call <vilib>:"Add State(s) to Queue__JKI_lib_State_Machine.vi"("State(s) in (\"\")"=w316) -> ("States Out"=w315:string)  [unwired: 14 in]
      }
    }
  }
